vi "FindServersInterface.vi"(0 "Servers":T2[](array[typedef]), 1 "Interface":T1) -> (2 "Found":bool, 3 "Server Index":i32, 4 "Interface Index":i32)   [LabVIEW 2017]
uses:
  <vilib>/WebServerConfig/Server.ctl
  <vilib>/WebServerConfig/Alias.ctl
  <vilib>/WebServerConfig/ErrorDocument.ctl
  <vilib>/WebServerConfig/Action.ctl
  <vilib>/WebServerConfig/Redirect.ctl
  <vilib>/WebServerConfig/Interface.ctl
  <vilib>/WebServerConfig/AddHandler.ctl
  <vilib>/WebServerConfig/SSL.ctl
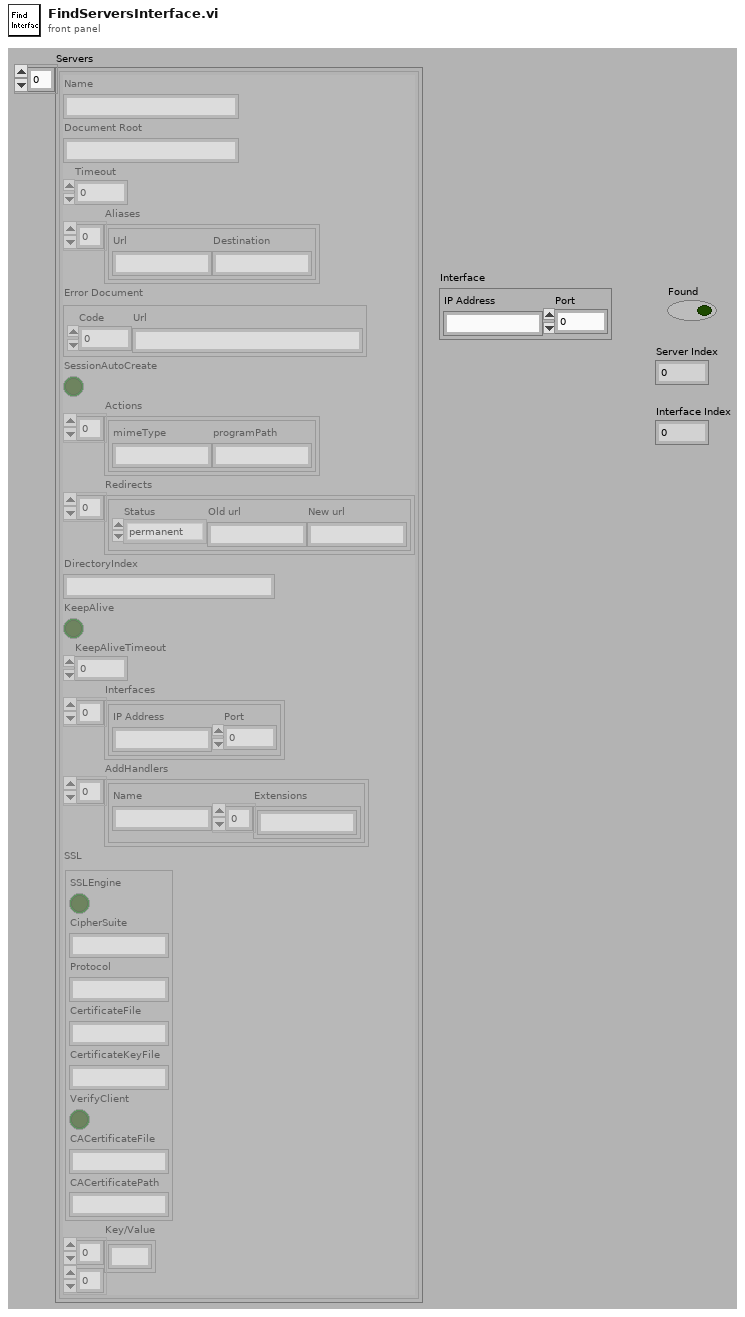
[diagram p1: front panel]
types:
  T1 = typedef "Interface.ctl" = cluster{"IP Address":string, "Port":u16}
  T2 = typedef "Server.ctl" = cluster{"Name":string, "Document Root":string, "Timeout":u32, "Aliases":T3[], "Error Document":T4, "SessionAutoCreate":bool, "Actions":T5[], "Redirects":T6[], "DirectoryIndex":string, "KeepAlive":bool, "KeepAliveTimeout":u32, "Interfaces":T1[], "AddHandlers":T7[], "SSL":T8, "Key/Value":string[][]}
  T3 = typedef "Alias.ctl" = cluster{"Url":string, "Destination":string}
  T4 = typedef "ErrorDocument.ctl" = cluster{"Code":u16, "Url":string}
  T5 = typedef "Action.ctl" = cluster{"mimeType":string, "programPath":string}
  T6 = typedef "Redirect.ctl" = cluster{"Status":enum16{"permanent", "temp", "seeother", "gone"}, "Old url":string, "New url":string}
  T7 = typedef "AddHandler.ctl" = cluster{"Name":string, "Extensions":string[]}
  T8 = typedef "SSL.ctl" = cluster{"SSLEngine":bool, "CipherSuite":string, "Protocol":string, "CertificateFile":string, "CertificateKeyFile":string, "VerifyClient":bool, "CACertificateFile":string, "CACertificatePath":string}
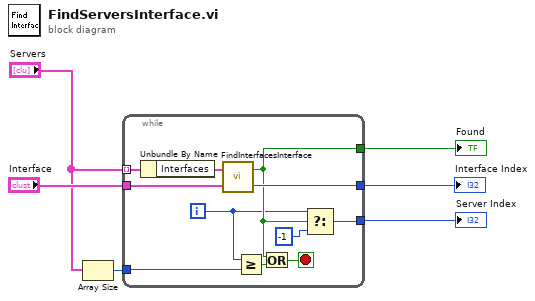
[diagram p0: block diagram]
diagram:
  n1 = Array Size(array="Servers") -> (size(s)=w1:i32)
  n2 = while {
    tunnel: "Interface" -> [w17]
    tunnel: "Servers" -> [w15] mode=indexing
    tunnel: [w10] -> w5
    tunnel: [w16] -> w6
    tunnel: [w8] -> w3
    tunnel: w1 -> [w13]
    i -> [w9]
    stop <- w11 stop-if-true
    n3 = Unbundle By Name(w15) -> ("Interfaces"=w14:T1[])
    n4 = call <vilib>:"FindInterfacesInterface.vi"("Interface"=w17, "Interfaces"=w14) -> ("Index"=w16:i32, "Found"=w10:bool)
    n5 = Greater Or Equal?(x=w9, y=w13) -> (x >= y?=w12:bool)
    n6 = Or(x=w10, y=w12) -> (x .or. y?=w11:bool)
    n7 = Select(t=w9, s=w10, f=-1) -> (s? t:f=w8:i32)
  }
  "Interface Index" <- w6
  "Server Index" <- w3
  "Found" <- w5
